vi "FPGA Main (Container).vi"   [LabVIEW 2025]
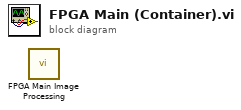
[diagram p0: block diagram]
diagram:
  n1 = call "FPGA Main Image Processing.vi"() -> ()  [unwired: 12 in]
